vi "Configure.vi"(8 "error in (no error)":errorcluster, 11 "TomoConversion in":refnum<class "TomoConversion.lvclass">) -> (0 "error out":errorcluster, 2 "cancelled?":bool, 3 "TomoConversion out":refnum<class "TomoConversion.lvclass">)   [LabVIEW 2012, in "TomoConversion.lvclass"]
doc: "The configure method configures the details for the RabbitMQ connection. \n\nIn the derived class, make a call to the parent for setting these parameters."
uses:
  TomoConversion.lvclass
  <vilib>/Utility/miscctls.llb/LVPointTypeDef.ctl
  TomoConversion.lvclass/TomoConversion.ctl
  <vilib>/Distrio/Murmex/Murmex/Murmex.lvclass
panel:
  in  "button::cancel":bool
  in  "button::configuremurmex":bool
  in  "button::ok":bool
  in  "auxiliary director path":path
  in  "conversion directory path":path
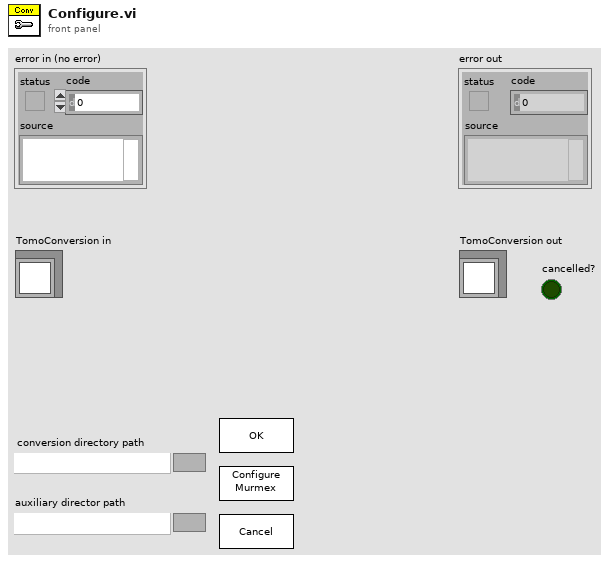
[diagram p1: front panel]
types:
  T1 = typedef "LVPointTypeDef.ctl" = cluster{"Horizontal":i16, "Vertical":i16}
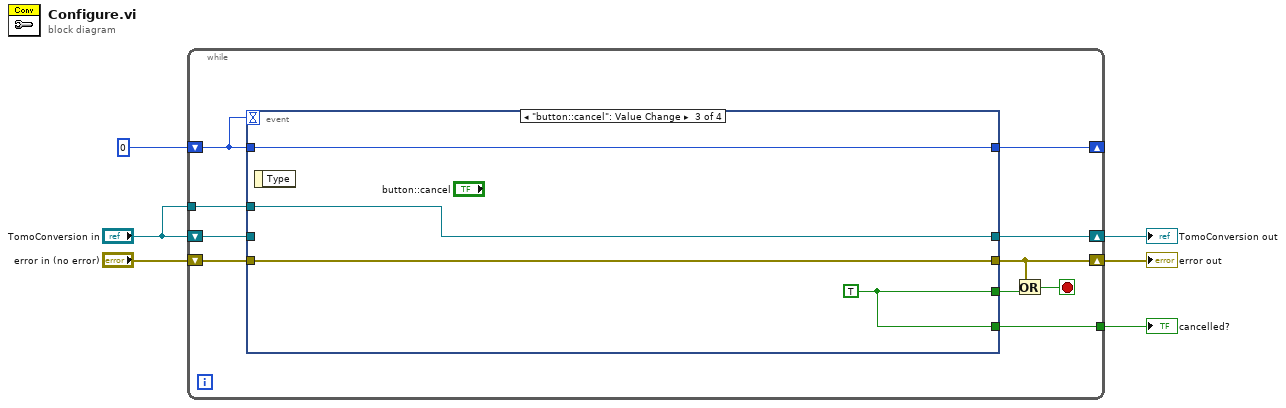
[diagram p0: block diagram]
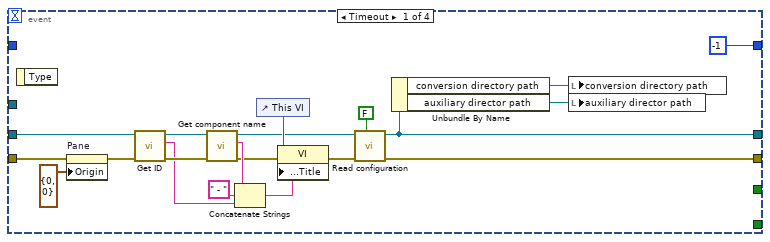
[diagram p2: hidden frame]
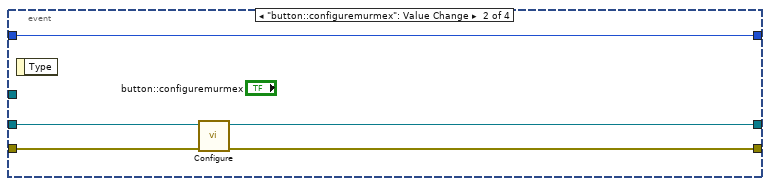
[diagram p3: hidden frame]
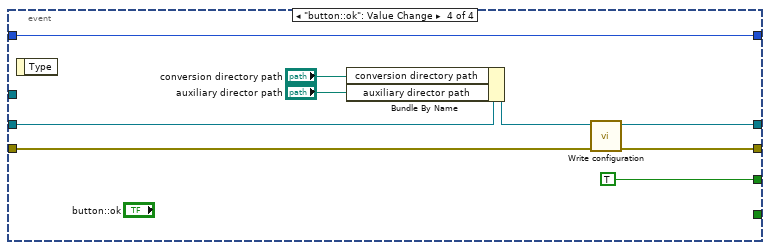
[diagram p4: hidden frame]
diagram:
  n1 = while {
    shift-right: [w11] -> _
    shift-left: 0 -> [w16]
    shift-right: [w12] -> w1
    shift-left: "TomoConversion in" -> [w14]
    shift-right: [w9] -> w2
    shift-left: "error in (no error)" -> [w13]
    tunnel: "TomoConversion in" -> [w15]
    tunnel: [w10] -> w3
    stop <- w7 stop-if-true
    n2 = event shown="[2] \"button::cancel\": Value Change" {
      selector: _ -> [_ _ _ _]
      dyn-events: _ -> [_ _ _ _]
      timeout: w16 -> [_ _ _ _]
      tunnel: w16 -> [_ w37 w42 w46]
      tunnel: w15 -> [_ _ w44 _]
      tunnel: w14 -> [w33 w40 _ w54]
      tunnel: w13 -> [w36 w41 w45 w51]
      tunnel: [w21 w38 w45 w50] -> w9
      tunnel: [w20 w39 w44 w52] -> w12
      tunnel: [-1 w37 w42 w46] -> w11
      tunnel: [_ _ w43 TRUE] -> w8
      tunnel: [_ _ w43 _] -> w10
      event Timeout {
        n3 = event-data() -> ()  [unwired: 1 in, 1 out]
        n4 = property on="Pane" class="Pane"(error in=w36, "Origin"=T1 {"Horizontal"=0, "Vertical"=0}) -> (error out=w34:errorcluster)  [unwired: 1 in, 1 out]
        n5 = call <vilib>:"Get ID.vi"("error in (no error)"=w34, "Murmex in"=w33) -> ("error out"=w31:errorcluster, "component id"=w29:string, "Murmex out"=w32:refnum<class "TomoConversion.lvclass">)  [unwired: 7 in]
        n6 = call <vilib>:"Get component name.vi"("error in (no error)"=w31, "Murmex in"=w32) -> ("error out"=w27:errorcluster, "component name"=w30:string, "Murmex out"=w23:refnum<class "TomoConversion.lvclass">)  [unwired: 7 in]
        n7 = Concatenate Strings(w30, " - " ("string"), w29) -> (w25:string)
        n8 = control-ref of="This VI"() -> (w26:refnum<vi>)
        n9 = property class="VI"(reference=w26, error in=w27, "Front Panel.Title"=w25) -> (error out=w24:errorcluster)  [unwired: 1 out]
        n10 = call-dynamic "Read configuration.vi"("force loading?"=FALSE, "error in (no error)"=w24, "TomoConversion in"=w23) -> ("error out"=w21:errorcluster, "TomoConversion out"=w20:refnum<class "TomoConversion.lvclass">)  [unwired: 7 in]
        n11 = Unbundle By Name(w20) -> ("conversion directory path"=w19:path, "auxiliary director path"=w18:path)
        n12 = local write "conversion directory path"(w19) -> ()
        n13 = local write "auxiliary director path"(w18) -> ()
      }
      event "button::configuremurmex": Value Change {
        n14 = event-data() -> ()  [unwired: 1 in, 1 out]
        n15 = call-parent "Configure.vi"("error in (no error)"=w41, "Murmex in"=w40) -> ("error out"=w38:errorcluster, "Murmex out"=w39:refnum<class "TomoConversion.lvclass">)  [unwired: 7 in, 1 out]
      }
      event "button::cancel": Value Change {
        w43 = TRUE
        n16 = event-data() -> ()  [unwired: 1 in, 1 out]
      }
      event "button::ok": Value Change {
        n17 = event-data() -> ()  [unwired: 1 in, 1 out]
        n18 = Bundle By Name(cluster=w54, "conversion directory path"="conversion directory path", "auxiliary director path"="auxiliary director path") -> (w53:refnum<class "TomoConversion.lvclass">)
        n19 = call-dynamic "Write configuration.vi"("error in (no error)"=w51, "TomoConversion in"=w53) -> ("error out"=w50:errorcluster, "TomoConversion out"=w52:refnum<class "TomoConversion.lvclass">)  [unwired: 8 in]
      }
    }
    n20 = Or(x=w9, y=w8) -> (x .or. y?=w7:bool)
  }
  "error out" <- w2
  "TomoConversion out" <- w1
  "cancelled?" <- w3
